vi "Setting Database.Refresh.Synchronous.vi"(6 "Timeout":i32, 8 "error in (no error)":errorcluster, 10 "Initialize":T6, 11 "Setting Database in":refnum<class "Setting Database.lvclass">) -> (0 "error out":errorcluster, 2 "Response":T5, 3 "Setting Database out":refnum<class "Setting Database.lvclass">)   [LabVIEW 2019, in "Setting Database.lvclass"]
uses:
  Setting Database.lvclass
  Typedefs/PrivateEvents--Setting Database.Refresh.ctl
  Typedefs/PublicEvents--Setting Database.PathsUpdated.ctl
  Path Settings/Path Settings.lvclass
  Typedefs/PublicEvents--Setting Database.RectanglesUpdated.ctl
  Rectangle Settings/Rectangle Settings.lvclass
  Typedefs/PublicEvents--Setting Database.FunnelsUpdated.ctl
  Funnel Settings/Funnel Settings.lvclass
  Typedefs/PublicEvents--Setting Database.DotsUpdated.ctl
  Dot Settings/Dot Settings.lvclass
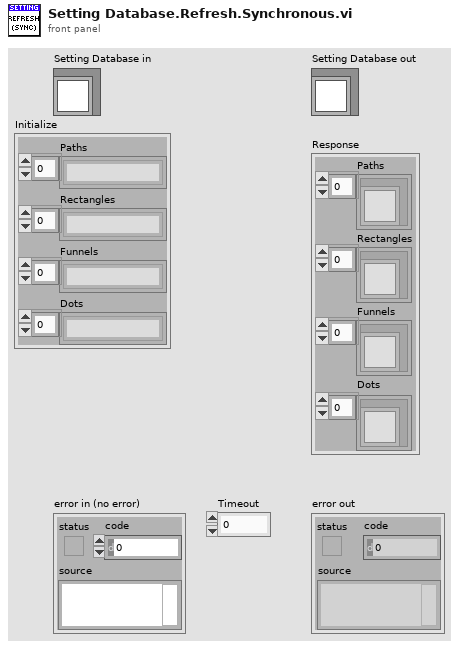
[diagram p1: front panel]
types:
  T1 = typedef "Setting Database.lvclass/PublicEvents--Setting Database.PathsUpdated.ctl" = refnum<class "Path Settings.lvclass">[]
  T2 = typedef "Setting Database.lvclass/PublicEvents--Setting Database.RectanglesUpdated.ctl" = refnum<class "Rectangle Settings.lvclass">[]
  T3 = typedef "Setting Database.lvclass/PublicEvents--Setting Database.FunnelsUpdated.ctl" = refnum<class "Funnel Settings.lvclass">[]
  T4 = typedef "Setting Database.lvclass/PublicEvents--Setting Database.DotsUpdated.ctl" = refnum<class "Dot Settings.lvclass">[]
  T5 = cluster{"Paths":T1, "Rectangles":T2, "Funnels":T3, "Dots":T4}
  T6 = typedef "Setting Database.lvclass/PrivateEvents--Setting Database.Refresh.ctl" = cluster{"Paths":string[], "Rectangles":string[], "Funnels":string[], "Dots":string[]}
  T7 = typedef "Setting Database.lvclass/PublicEvents--Cluster.ctl" = cluster{"NewActivePath":refnum<user-event>, "PathsUpdated":refnum<user-event>, "RectanglesUpdated":refnum<user-event>, "NewActiveRectangle":refnum<user-event>, "NewActiveFunnel":refnum<user-event>, "FunnelsUpdated":refnum<user-event>, "NewActiveDot":refnum<user-event>, "DotsUpdated":refnum<user-event>}
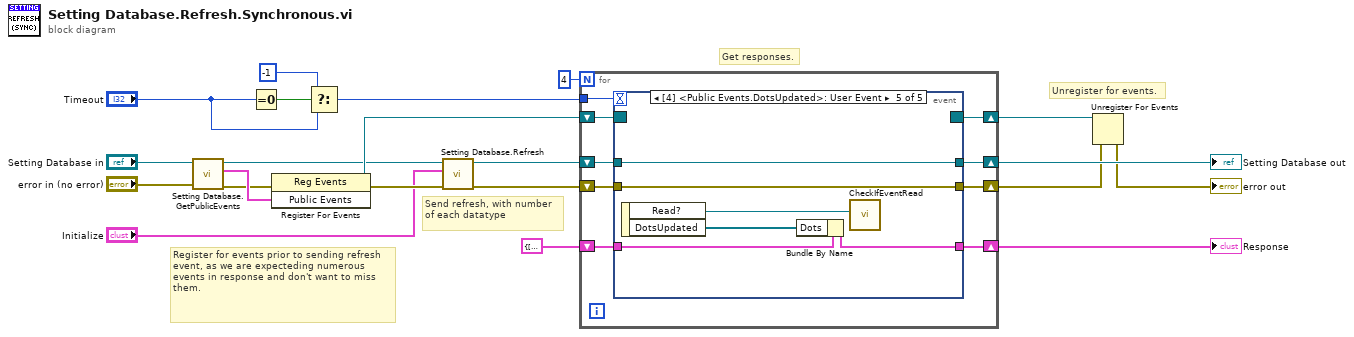
[diagram p0: block diagram]
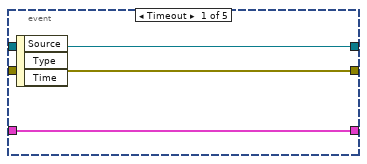
[diagram p2: hidden frame]
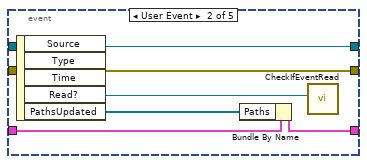
[diagram p3: hidden frame]
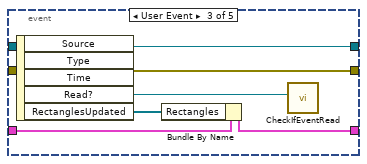
[diagram p4: hidden frame]
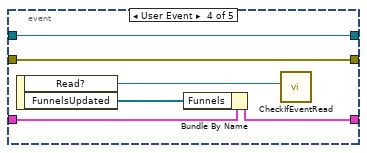
[diagram p5: hidden frame]
diagram:
  # "Unregister for events."
  # "Get responses."
  # "Send refresh, with number of each datatype"
  # "Register for events prior to sending refresh event, as we are expecteding numerous events in response and don't want to miss them."
  n1 = call "Setting Database.GetPublicEvents.vi"("error in (no error)"="error in (no error)", "Setting Database"="Setting Database in") -> ("error out"=w18:errorcluster, "Public Events"=w19:T7, "Setting Database out"=w15:refnum<class "Setting Database.lvclass">)  [unwired: 7 in]
  n2 = Equal To 0?(x="Timeout") -> (x = 0?=w4:bool)
  n3 = register-events(error in=w18, w19) -> (reference out=w16:refnum<event-registration>, error out=w13:errorcluster)  [unwired: 1 in]
  n4 = Select(t=-1, s=w4, f="Timeout") -> (s? t:f=w1:i32)
  n5 = call "Setting Database.Refresh.vi"("error in (no error)"=w13, "Initialize"="Initialize", "Setting Database"=w15) -> ("error out"=w12:errorcluster, "Setting Database out"=w14:refnum<class "Setting Database.lvclass">)  [unwired: 7 in]
  n6 = for {
    N: 4 -> [_]
    shift-right: [w26] -> w10
    shift-left: w16 -> [w29]
    shift-right: [w30] -> w17
    shift-left: w14 -> [w28]
    shift-right: [w25] -> w8
    shift-left: w12 -> [w27]
    shift-right: [w23] -> w5
    shift-left: T5 {"Paths"=[], "Rectangles"=[], "Funnels"=[], "Dots"=[]} -> [w24]
    tunnel: w1 -> [w22]
    n7 = event shown="[4] <Public Events.DotsUpdated>: User Event" {
      selector: w29 -> [_ _ _ _ _]
      dyn-events: [_ _ _ _ _] -> w26
      timeout: w22 -> [_ _ _ _ _]
      tunnel: w28 -> [w33 w39 w45 w51 w52]
      tunnel: [w33 w39 w45 w51 w52] -> w30
      tunnel: [w32 w38 w44 w50 w57] -> w25
      tunnel: w27 -> [w32 w38 w44 w50 w57]
      tunnel: w24 -> [w31 w37 w43 w48 w55]
      tunnel: [w31 w36 w41 w47 w54] -> w23
      event Timeout {
        n8 = event-data() -> ()  [unwired: 1 in, 3 out]
      }
      event User Event {
        n9 = event-data() -> ("Read?"=w34:refnum<notifier>, "PathsUpdated"=w35:T1)  [unwired: 1 in, 3 out]
        n10 = Bundle By Name(cluster=w37, "Paths"=w35) -> (w36:T5)
        n11 = call "CheckIfEventRead.vi"("Read?"=w34) -> ()  [unwired: 9 in, 2 out]
      }
      event User Event {
        n12 = event-data() -> ("Read?"=w40:refnum<notifier>, "RectanglesUpdated"=w42:T2)  [unwired: 1 in, 3 out]
        n13 = Bundle By Name(cluster=w43, "Rectangles"=w42) -> (w41:T5)
        n14 = call "CheckIfEventRead.vi"("Read?"=w40) -> ()  [unwired: 9 in, 2 out]
      }
      event User Event {
        n15 = event-data() -> ("Read?"=w46:refnum<notifier>, "FunnelsUpdated"=w49:T3)  [unwired: 1 in]
        n16 = Bundle By Name(cluster=w48, "Funnels"=w49) -> (w47:T5)
        n17 = call "CheckIfEventRead.vi"("Read?"=w46) -> ()  [unwired: 9 in, 2 out]
      }
      event User Event {
        n18 = event-data() -> ("Read?"=w53:refnum<notifier>, "DotsUpdated"=w56:T4)  [unwired: 1 in]
        n19 = Bundle By Name(cluster=w55, "Dots"=w56) -> (w54:T5)
        n20 = call "CheckIfEventRead.vi"("Read?"=w53) -> ()  [unwired: 9 in, 2 out]
      }
    }
  }
  "Setting Database out" <- w17
  "Response" <- w5
  n21 = Unregister For Events(event registration refnum=w10, error in=w8) -> (error out=→"error out":errorcluster)
